vi "Write Result Data.vi"(8 "error in (no error)":errorcluster, 10 "Result Data":T1, 11 "Test Result in":refnum<class "Test Result.lvclass">) -> (0 "error out":errorcluster, 3 "Test Result out":refnum<class "Test Result.lvclass">)   [LabVIEW 2021, in "Sequence Engine.lvlib" / "Test Result.lvclass"]
uses:
  Test Result.lvclass
  Result Data.ctl
  Test Status.ctl
  Test Result.lvclass/Test Result.ctl
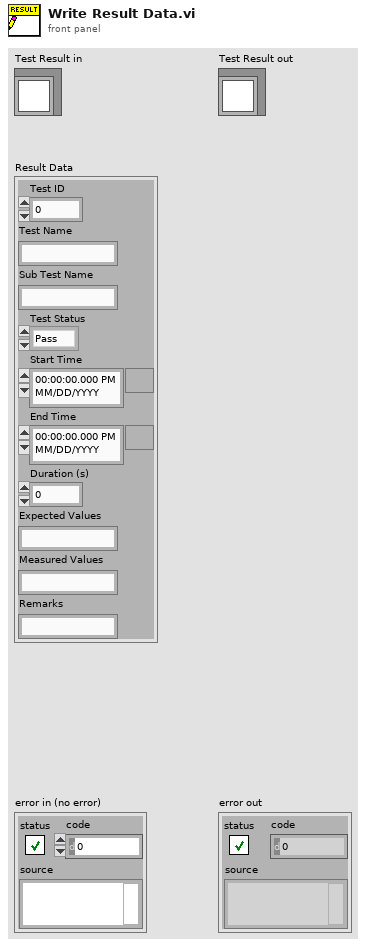
[diagram p1: front panel]
types:
  T1 = typedef "Sequence Engine.lvlib/Test Result.lvclass/Result Data.ctl" = cluster{"Test ID":u32, "Test Name":string, "Sub Test Name":string, "Test Status":T2, "Start Time":timestamp, "End Time":timestamp, "Duration (s)":dbl, "Expected Values":string, "Measured Values":string, "Remarks":string}
  T2 = typedef "Sequence Engine.lvlib/Test Result.lvclass/Test Status.ctl" = enum16{"Pass", "Fail", "Aborted", "Skipped"}
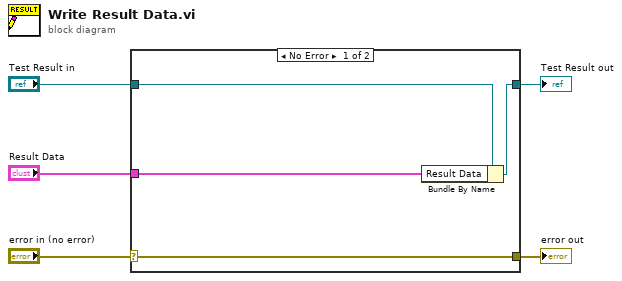
[diagram p0: block diagram]
diagram:
  n1 = case shown="No Error" "error in (no error)" {
    selector: "error in (no error)" -> [w9 w10]
    tunnel: [w9 w10] -> w4
    tunnel: [w7 w11] -> w2
    tunnel: "Test Result in" -> [w8 w11]
    tunnel: "Result Data" -> [w6 _]
    frame No Error {
      n2 = Bundle By Name(cluster=w8, "Result Data"=w6) -> (w7:refnum<class "Test Result.lvclass">)
    }
    frame Error {
    }
  }
  "error out" <- w4
  "Test Result out" <- w2
